vi "Delete Error.vi"(8 "error in (no error)":errorcluster, 11 "[error code] (0)":i32 format="%0.0f") -> (0 "error out":errorcluster)   [LabVIEW 2014, in "Utilities.lvlib"]
uses:
  Utilities.lvlib
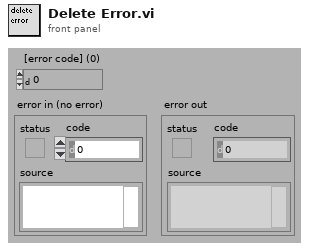
[diagram p1: front panel]
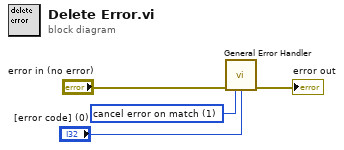
[diagram p0: block diagram]
diagram:
  w1 = 1 items=["no exception", "cancel error on match", "set error on match"] ("[exception action] (none:0)")
  n1 = call <vilib>:"General Error Handler.vi"("error in (no error)"="error in (no error)", "[exception action] (none:0)"=w1, "[exception code]"="[error code] (0)") -> ("error out"=→"error out":errorcluster)  [unwired: 8 in, 4 out]
